vi "PVCAM_GetCameraName.vi"(8 "error in (no error)":errorcluster, 11 "index in":i16) -> (0 "error out":errorcluster, 1 "cameraName array":u8[](array[numeric]), 2 "return out":i16, 3 "string":string)   [LabVIEW 2021]
uses:
  pvcam64.dll
panel:
  out "index out":i16
  in  "return in":i16
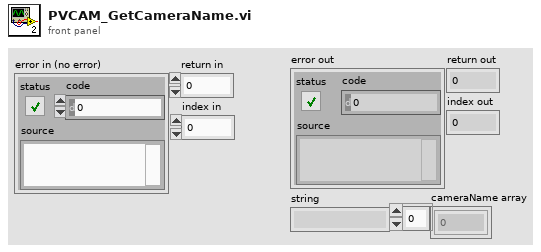
[diagram p1: front panel]
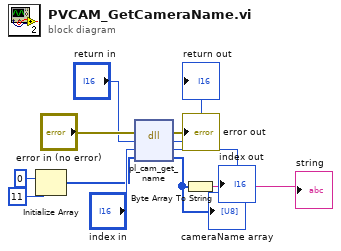
[diagram p0: block diagram]
diagram:
  n1 = Initialize Array(u8 0 ("element"), 11 ("dimension size")) -> (w2:u8[])
  n2 = dll-call lib="pvcam64.dll" fn="pl_cam_get_name"(error in="error in (no error)", "return type"="return in", "index"="index in", "cameraName"=w2) -> (error out=→"error out":errorcluster, "return type"=→"return out":i16, "index"=→"index out":i16, "cameraName"=w3:u8[])  [unwired: 1 in, 1 out]
  "cameraName array" <- w3
  n3 = Byte Array To String(unsigned byte array=w3) -> (string=→"string":string)
